vi "HTML Report Token Converter.vi"(1 "String In":string) -> (0 "String Out":string)   [LabVIEW 2020, in "NI_ReportGenerationCore.lvlib"]
uses:
  <vilib>/Utility/NIReport.llb/NI_ReportGenerationCore.lvlib
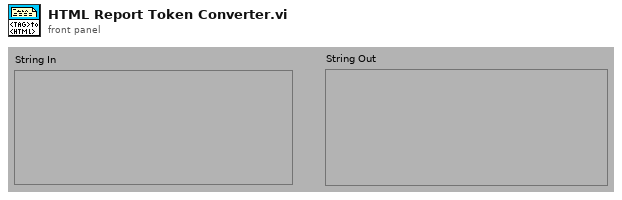
[diagram p1: front panel]
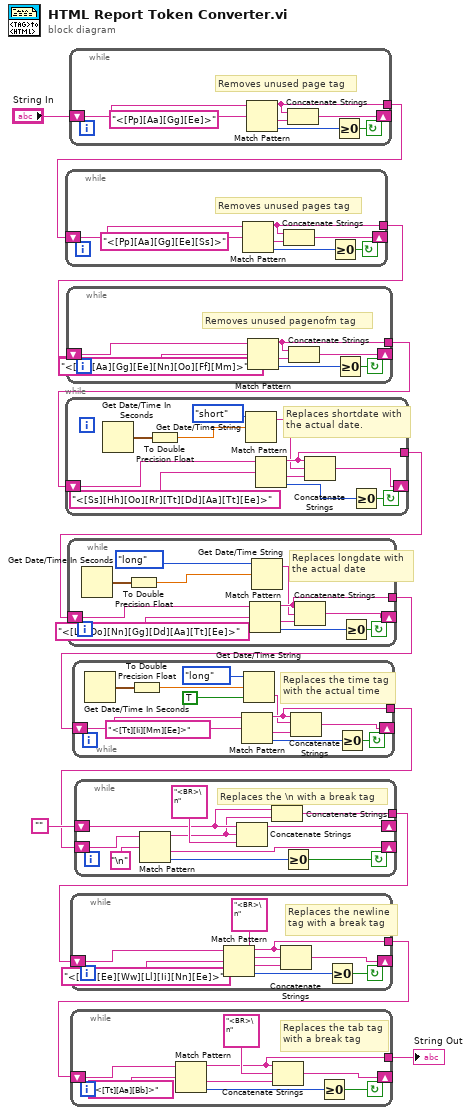
[diagram p0: block diagram]
diagram:
  n1 = while {
    tunnel: [w12] -> w7
    shift-left: "String In" -> [w14]
    shift-right: [w15] -> _
    stop <- w13 continue-if-true
    # "Removes unused page tag"
    n2 = Match Pattern(string=w14, regular expression="<[Pp][Aa][Gg][Ee]>") -> (before substring=w12:string, after substring=w17:string, offset past match=w16:i32)  [unwired: 2 out]
    n3 = Concatenate Strings(w12, w17) -> (w15:string)
    n4 = Greater Or Equal To 0?(x=w16) -> (x >= 0?=w13:bool)
  }
  n5 = while {
    tunnel: [w19] -> w8
    shift-left: w7 -> [w21]
    shift-right: [w22] -> _
    stop <- w20 continue-if-true
    # "Removes unused pages tag"
    n6 = Match Pattern(string=w21, regular expression="<[Pp][Aa][Gg][Ee][Ss]>") -> (before substring=w19:string, after substring=w24:string, offset past match=w23:i32)  [unwired: 2 out]
    n7 = Concatenate Strings(w19, w24) -> (w22:string)
    n8 = Greater Or Equal To 0?(x=w23) -> (x >= 0?=w20:bool)
  }
  n9 = while {
    tunnel: [w26] -> w10
    shift-left: w8 -> [w28]
    shift-right: [w29] -> _
    stop <- w27 continue-if-true
    # "Removes unused pagenofm tag"
    n10 = Match Pattern(string=w28, regular expression="<[Pp][Aa][Gg][Ee][Nn][Oo][Ff][Mm]>") -> (before substring=w26:string, after substring=w31:string, offset past match=w30:i32)  [unwired: 2 out]
    n11 = Concatenate Strings(w26, w31) -> (w29:string)
    n12 = Greater Or Equal To 0?(x=w30) -> (x >= 0?=w27:bool)
  }
  n13 = while {
    tunnel: [w37] -> w9
    shift-left: w10 -> [w39]
    shift-right: [w40] -> _
    stop <- w38 continue-if-true
    # "Replaces shortdate with\nthe actual date."
    n14 = Get Date/Time In Seconds() -> (seconds since 1Jan1904=w34:timestamp)
    n15 = To Double Precision Float(number=w34) -> (double precision float=w33:dbl)
    n16 = Get Date/Time String(date format (0)=enum16{"short", "long", "abbreviated"}."short", seconds (now)=w33) -> (date string=w36:string)  [unwired: 1 in, 1 out]
    n17 = Match Pattern(string=w39, regular expression="<[Ss][Hh][Oo][Rr][Tt][Dd][Aa][Tt][Ee]>") -> (before substring=w37:string, after substring=w42:string, offset past match=w41:i32)  [unwired: 2 out]
    n18 = Concatenate Strings(w37, w36, w42) -> (w40:string)
    n19 = Greater Or Equal To 0?(x=w41) -> (x >= 0?=w38:bool)
  }
  n20 = while {
    tunnel: [w48] -> w6
    shift-left: w9 -> [w50]
    shift-right: [w51] -> _
    stop <- w49 continue-if-true
    # "Replaces longdate with\nthe actual date"
    n21 = Get Date/Time In Seconds() -> (seconds since 1Jan1904=w45:timestamp)
    n22 = To Double Precision Float(number=w45) -> (double precision float=w44:dbl)
    n23 = Match Pattern(string=w50, regular expression="<[Ll][Oo][Nn][Gg][Dd][Aa][Tt][Ee]>") -> (before substring=w48:string, after substring=w53:string, offset past match=w52:i32)  [unwired: 2 out]
    n24 = Get Date/Time String(date format (0)=enum16{"short", "long", "abbreviated"}."long", seconds (now)=w44) -> (date string=w47:string)  [unwired: 2 out]
    n25 = Concatenate Strings(w48, w47, w53) -> (w51:string)
    n26 = Greater Or Equal To 0?(x=w52) -> (x >= 0?=w49:bool)
  }
  n27 = while {
    tunnel: [w60] -> w4
    shift-left: w6 -> [w62]
    shift-right: [w63] -> _
    stop <- w61 continue-if-true
    # "Replaces the time tag\nwith the actual time"
    n28 = Get Date/Time In Seconds() -> (seconds since 1Jan1904=w56:timestamp)
    n29 = To Double Precision Float(number=w56) -> (double precision float=w55:dbl)
    n30 = Match Pattern(string=w62, regular expression="<[Tt][Ii][Mm][Ee]>") -> (before substring=w60:string, after substring=w65:string, offset past match=w64:i32)  [unwired: 2 out]
    n31 = Get Date/Time String(date format (0)=enum16{"short", "long", "abbreviated"}."long", seconds (now)=w55, want seconds? (F)=TRUE) -> (time string=w59:string)  [unwired: 1 out]
    n32 = Concatenate Strings(w60, w59, w65) -> (w63:string)
    n33 = Greater Or Equal To 0?(x=w64) -> (x >= 0?=w61:bool)
  }
  n34 = while {
    shift-left: "" ("Empty String Constant") -> [w69]
    shift-right: [w70] -> _
    tunnel: [w67] -> w1
    shift-left: w4 -> [w75]
    shift-right: [w71] -> _
    stop <- w74 continue-if-true
    # "Replaces the \\n with a break tag"
    n35 = Match Pattern(string=w75, regular expression="\n") -> (before substring=w68:string, after substring=w71:string, offset past match=w76:i32)  [unwired: 2 out]
    n36 = Concatenate Strings(w69, w68, "<BR>\n" ("Substring")) -> (w70:string)
    n37 = Concatenate Strings(w69, w68) -> (w67:string)
    n38 = Greater Or Equal To 0?(x=w76) -> (x >= 0?=w74:bool)
  }
  n39 = while {
    tunnel: [w77] -> w3
    shift-left: w1 -> [w79]
    shift-right: [w80] -> _
    stop <- w78 continue-if-true
    # "Replaces the newline\ntag with a break tag"
    n40 = Match Pattern(string=w79, regular expression="<[Nn][Ee][Ww][Ll][Ii][Nn][Ee]>") -> (before substring=w77:string, after substring=w83:string, offset past match=w81:i32)  [unwired: 2 out]
    n41 = Concatenate Strings(w77, "<BR>\n" ("Input 1"), w83) -> (w80:string)
    n42 = Greater Or Equal To 0?(x=w81) -> (x >= 0?=w78:bool)
  }
  n43 = while {
    tunnel: [w85] -> w2
    shift-left: w3 -> [w87]
    shift-right: [w88] -> _
    stop <- w86 continue-if-true
    # "Replaces the tab tag\nwith a break tag"
    n44 = Match Pattern(string=w87, regular expression="<[Tt][Aa][Bb]>") -> (before substring=w85:string, after substring=w91:string, offset past match=w89:i32)  [unwired: 2 out]
    n45 = Concatenate Strings(w85, "<BR>\n" ("Input 1"), w91) -> (w88:string)
    n46 = Greater Or Equal To 0?(x=w89) -> (x >= 0?=w86:bool)
  }
  "String Out" <- w2
